vi "P-733 XY Stage Engine.vi"(0 "Notifier Name":string, 11 "Axis Names":string[](array[string])) -> ()   [LabVIEW 2016]
uses:
  Microscope-Control-master/Microscope-Control-master/Device Library/Stages/Stages Controls/Stage Notifier Element.ctl
  Microscope-Control-master/Microscope-Control-master/Device Library/Stages/Stages Controls/Stage Actions.ctl
  Microscope-Control-master/Microscope-Control-master/Device Library/Stages/Stages Controls/Stage Status.ctl
  PI GCS2 DLL/PI_GCS2_DLL_x64.dll
panel:
  out "Success":u32
  in  "Right":bool
  in  "Left":bool
  in  "Y Position (µm)":dbl format="%#.3g"
  in  "Down":bool
  in  "Up":bool
  in  "X Position (µm)":dbl format="%#.3g"
  in  "Step Size (µm)":dbl=0.1
  in  "QUIT":bool
  in  "Abort":bool
  out "P-733 Found":bool
  out "Number Connected":i32
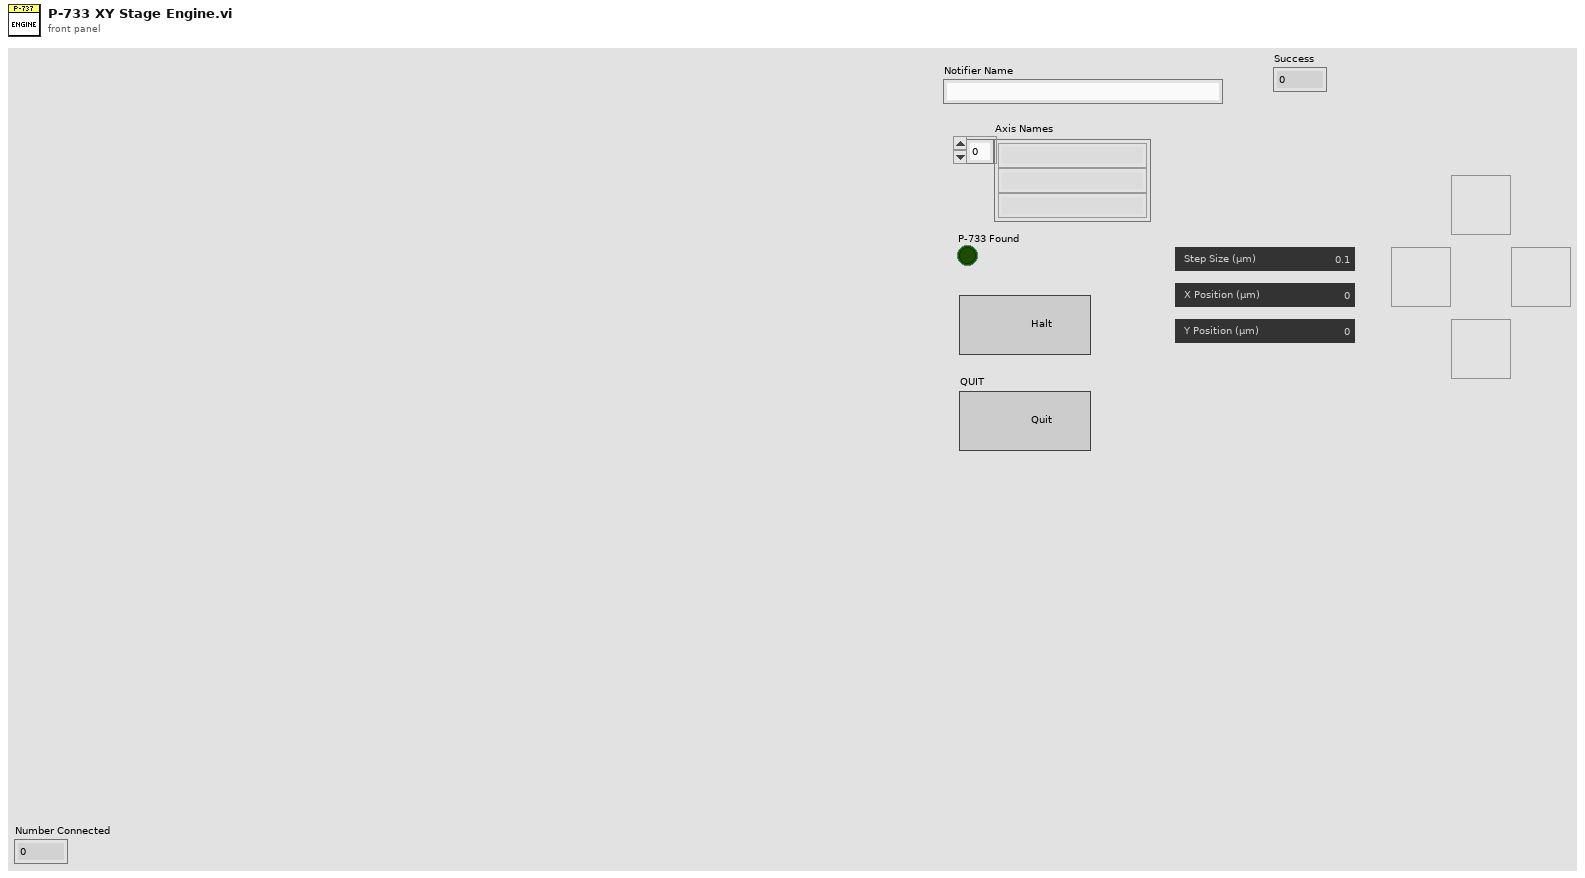
[diagram p1: front panel]
types:
  T1 = typedef "Stage Notifier Element.ctl" = cluster{"Action":T2, "Axis":bool[], "Setpoint":dbl[], "Velocity":dbl, "Cmd Recvd?":bool, "Position":dbl[], "Status":T3, "Misc":variant}
  T2 = typedef "Stage Actions.ctl" = enum16{"Get Position", "MVR", "MOVE", "HALT", "ONTARGET", "ERROR", "REFERENCE", "INIT", "VELOCITY", "STATUS", "EXIT", "HOME", "ZEROPOS", "NANOPOS", "ANALOG", "QUIT"}
  T3 = typedef "Stage Status.ctl" = enum16{"Error", "Abort", "Busy", "On Target"}
  T4 = enum32{"Invalid", "Standard", "Closed", "Hidden", "Minimized", "Maximized"}
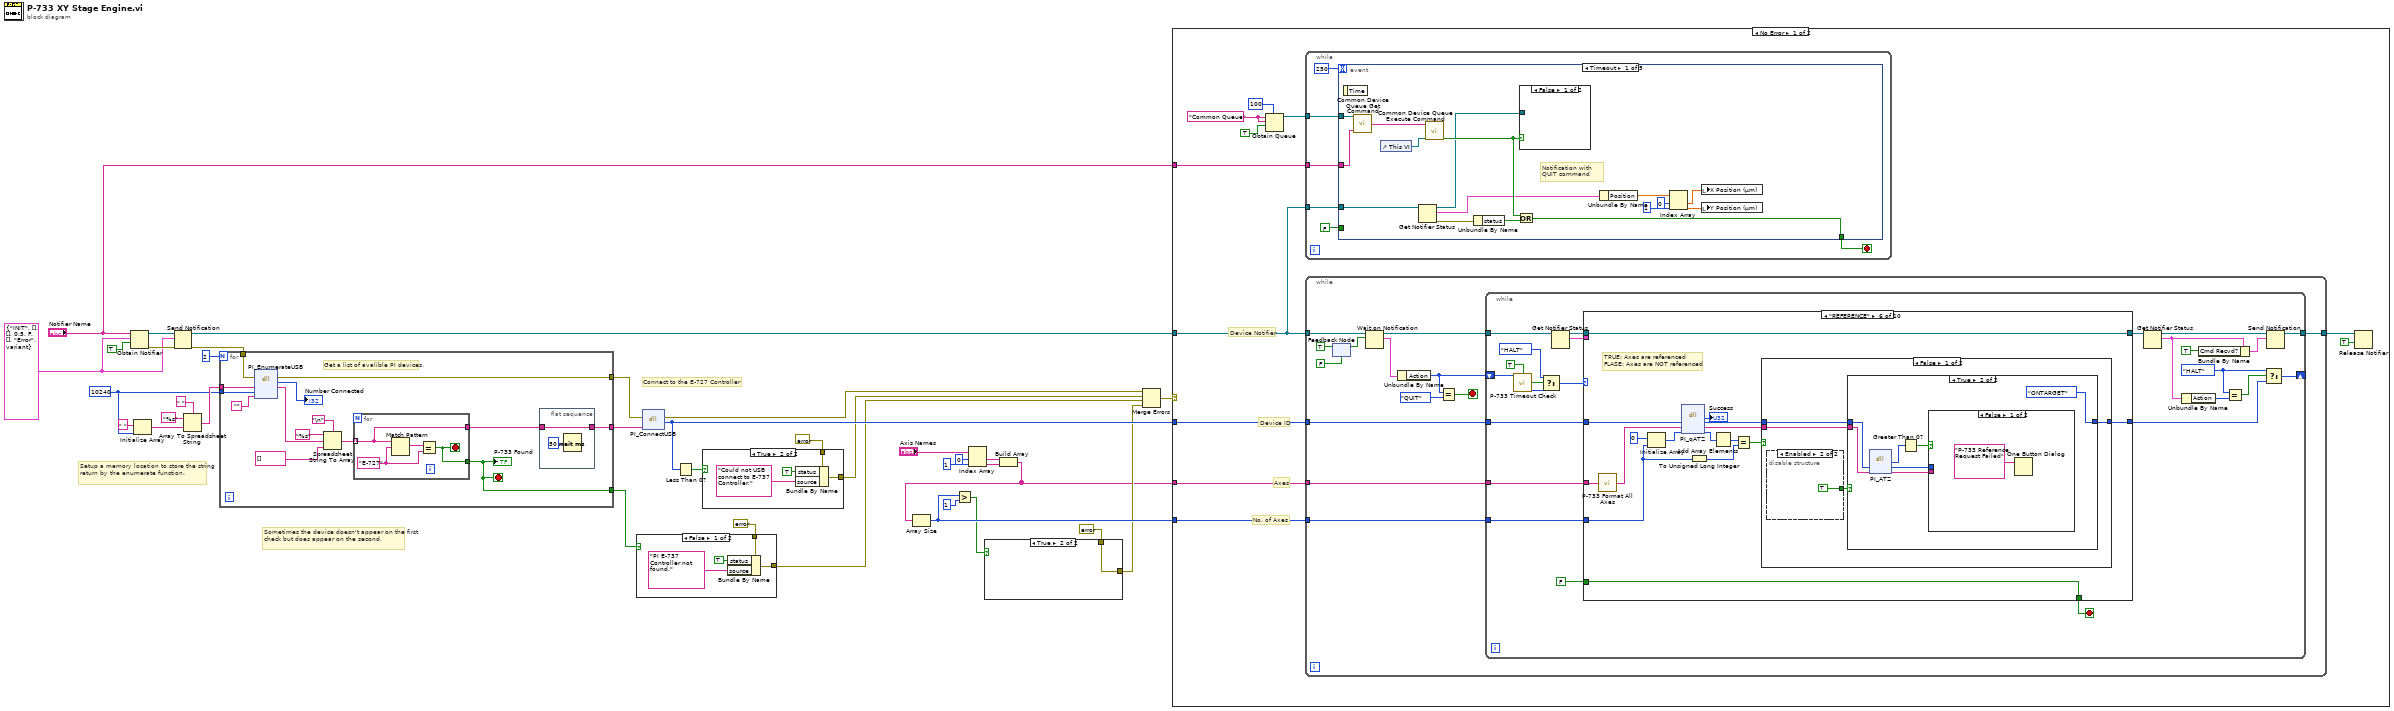
[diagram p0: block diagram]
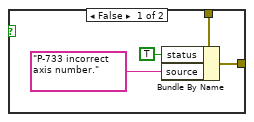
[diagram p2: hidden frame]
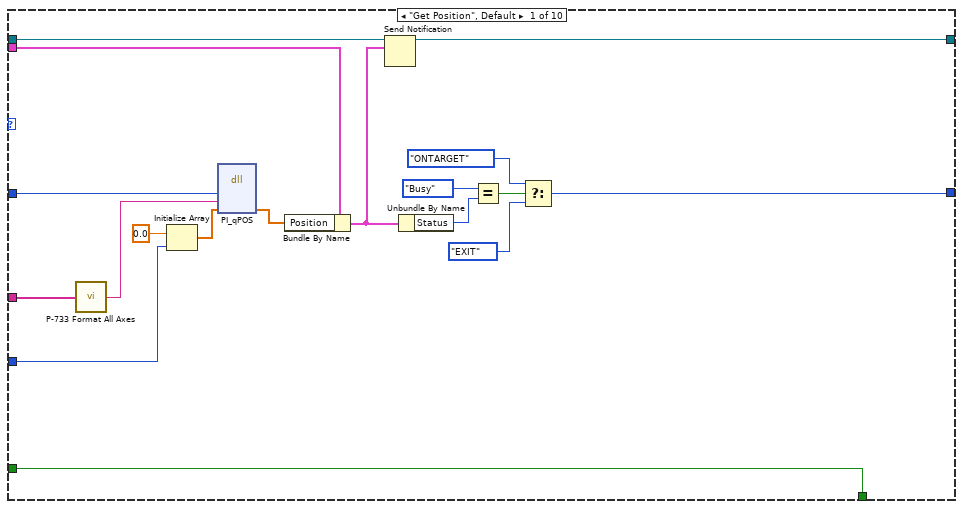
[diagram p5: hidden frame]
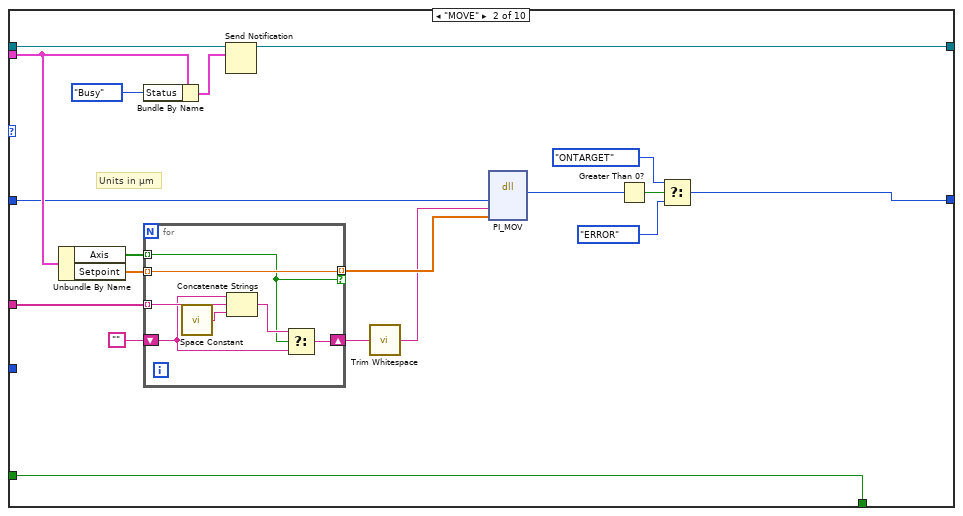
[diagram p6: hidden frame]
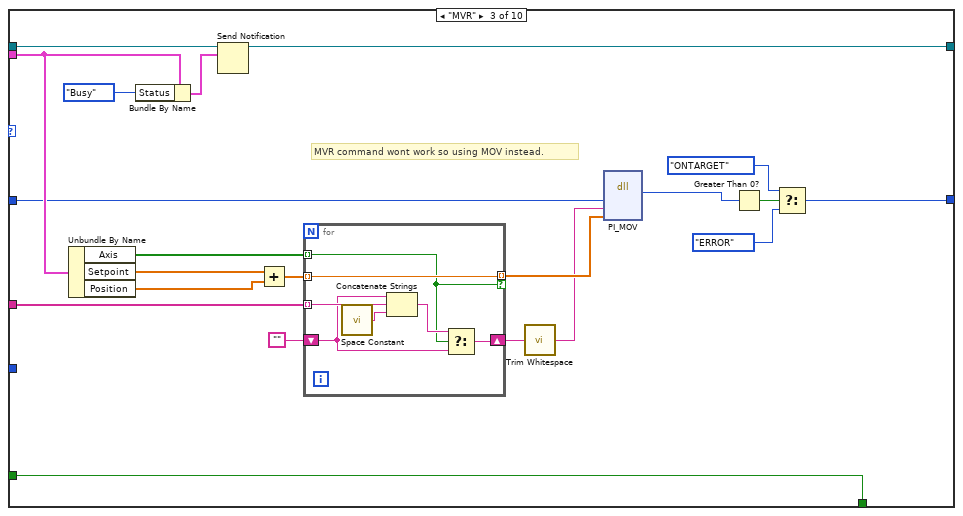
[diagram p7: hidden frame]
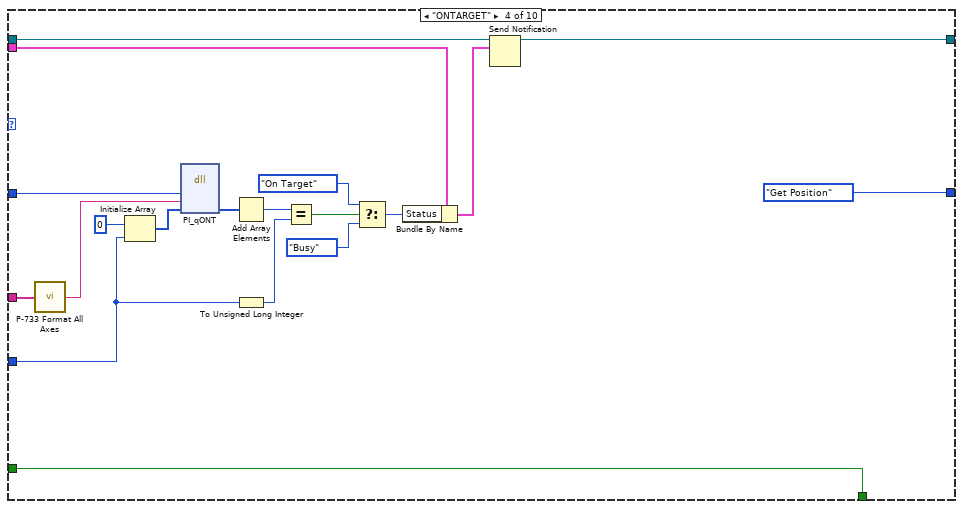
[diagram p8: hidden frame]
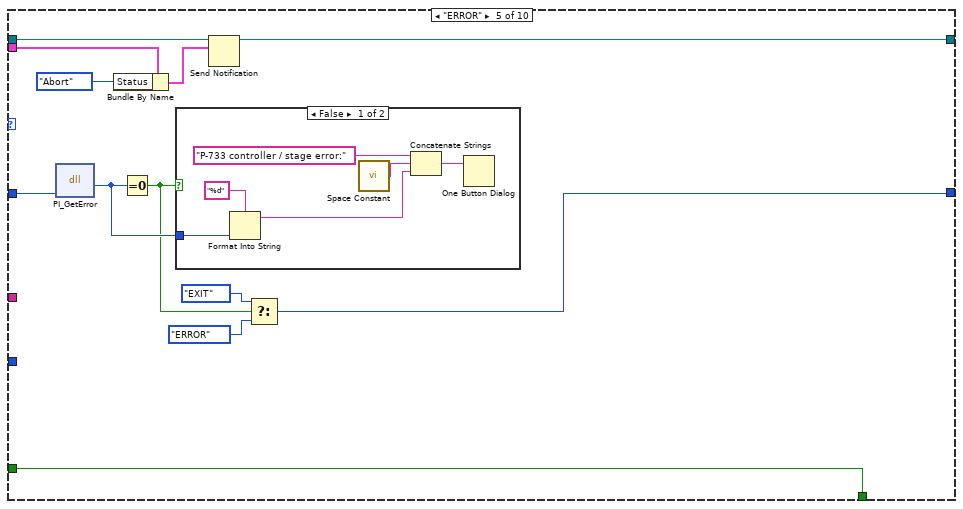
[diagram p9: hidden frame]
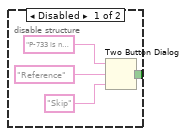
[diagram p11: hidden frame]
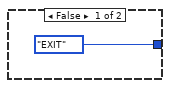
[diagram p12: hidden frame]
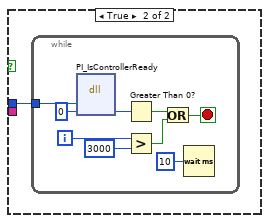
[diagram p13: hidden frame]
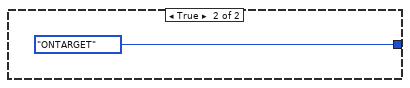
[diagram p14: hidden frame]
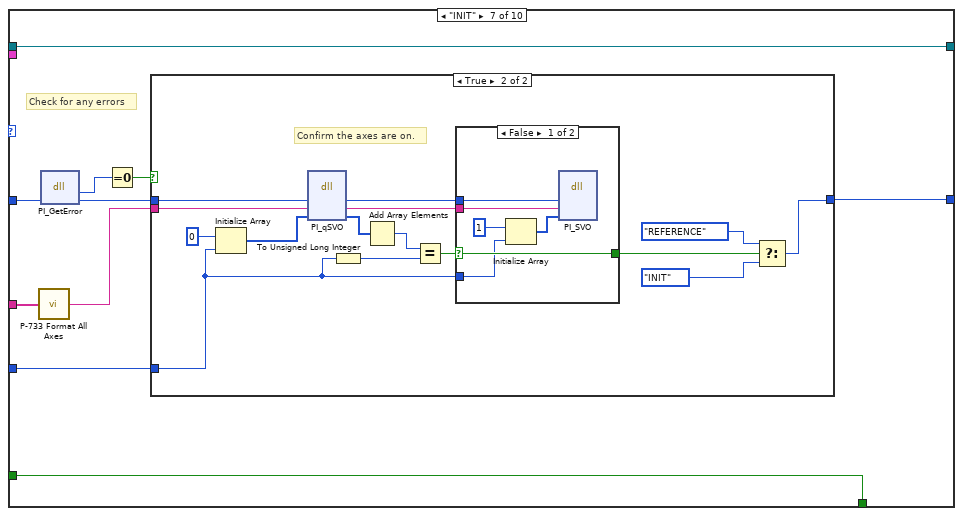
[diagram p15: hidden frame]
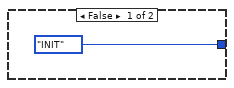
[diagram p16: hidden frame]
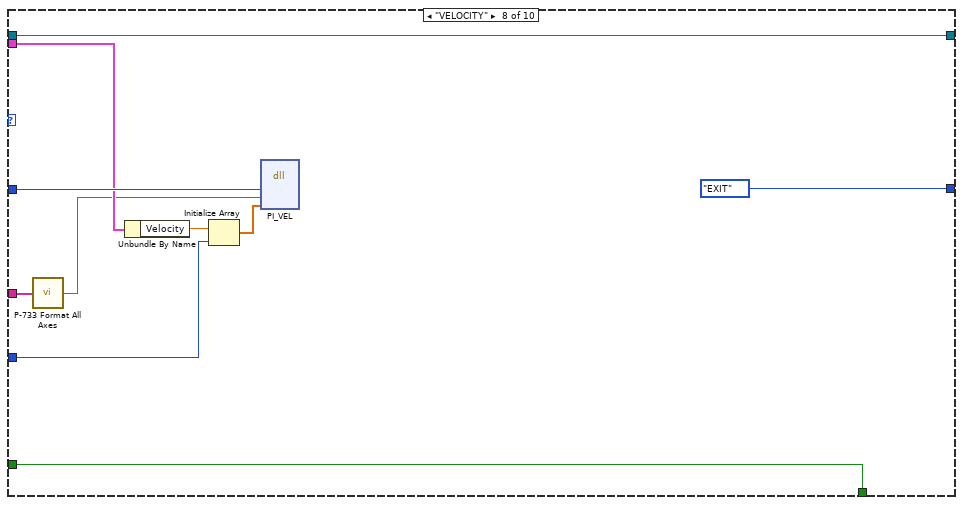
[diagram p18: hidden frame]
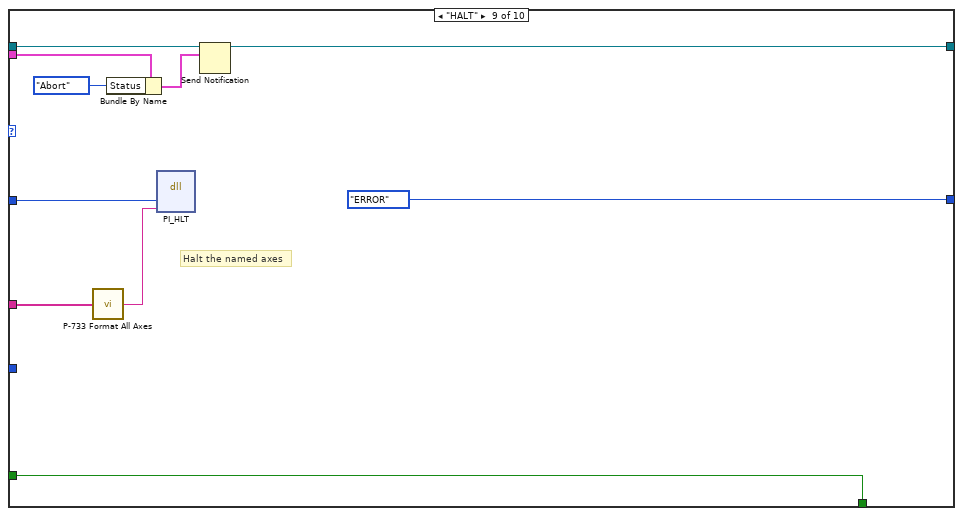
[diagram p19: hidden frame]
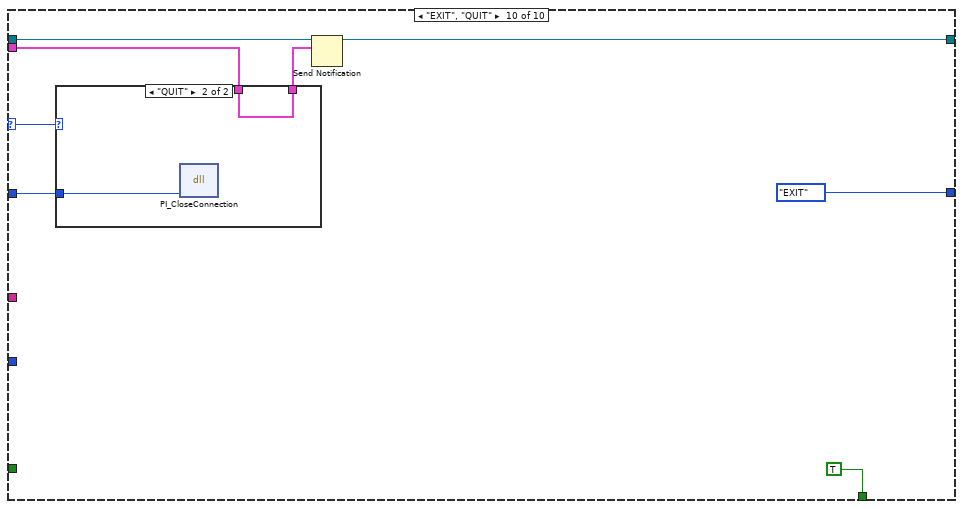
[diagram p20: hidden frame]
diagram:
  w14 = T1 {"Action"=enum."INIT", "Axis"=[], "Setpoint"=[], "Velocity"=0.5, "Cmd Recvd?"=FALSE, "Position"=[], "Status"=enum."Error", "Misc"=variant} ("Stage Status")
  w31 = 10240 ("dimension size")
  # "Setup a memory location to store the string return by the enumerate function."
  # "Connect to the E-727 Controller"
  # "Sometimes the device doesn't appear on the first check but does appear on the second."
  n1 = Obtain Notifier(name (unnamed)="Notifier Name", notification data type=w14, create if not found? (T)=TRUE) -> (notifier out=w17:refnum<notifier>, error out=w16:errorcluster)  [unwired: 1 in, 1 out]
  n2 = Initialize Array(" ", w31) -> (w35:string[])
  n3 = Send Notification(notification=w14, notifier=w17, error in (no error)=w16) -> (notifier out=w13:refnum<notifier>, error out=w15:errorcluster)
  n4 = Array To Spreadsheet String(delimiter (Tab)=" ", array=w35, 3:"%s" ("format string")) -> (spreadsheet string=w32:string)
  n5 = for {
    N: 2 -> [_]
    tunnel: w32 -> [w45]
    tunnel: w31 -> [w44]
    tunnel: [w40] -> w29
    tunnel: [w39] -> w23
    tunnel: [w38] -> w28
    tunnel: w15 -> [w37]
    stop <- w39 stop-if-true
    # "Get a list of avalible PI devices."
    n6 = dll-call lib="C:/Users/Ries Lab/Desktop/4Pi Labview/Microscope-Control/Device Library/Stages/PI/PI GCS2 DLL/PI_GCS2_DLL_x64.dll" fn="PI_EnumerateUSB"(error in=w37, "szBuffer"=w45, "iBufferSize"=w44, "szFilter"="") -> (error out=w38:errorcluster, "return type"=→"Number Connected":i32, "szBuffer"=w42:string)  [unwired: 4 in, 1 out]
    n7 = Spreadsheet String To Array(delimiter (Tab)="\n", format string="%s", spreadsheet string=w42, array type (2D Dbl)=string[] []) -> (array=w47:string[])
    n8 = for {
      tunnel: w47 -> [w54] mode=indexing
      tunnel: [w54] -> w41
      tunnel: [w53] -> w39
      stop <- w53 stop-if-true
      w55 = "E-727"
      n9 = Match Pattern(string=w54, regular expression=w55) -> (match substring=w56:string)  [unwired: 1 in, 3 out]
      n10 = Equal?(x=w56, y=w55) -> (x = y?=w53:bool)
    }
    "P-733 Found" <- w39
    n11 = flat-sequence {
      tunnel: w41 -> [w52]
      tunnel: [w52] -> w40
      frame #0 {
        n12 = Wait (ms)(milliseconds to wait=u32 50) -> ()  [unwired: 1 out]
      }
    }
  }
  n13 = case shown="False" w23 {
    tunnel: errorcluster {"status"=FALSE, "code"=0, "source"=""} ("error in (no error)") -> [w58 w61]
    tunnel: [w57 w61] -> w19
    frame False {
      n14 = Bundle By Name(cluster=w58, "status"=TRUE, "source"="PI E-737 Controller not found.") -> (w57:errorcluster)
    }
    frame True {
    }
  }
  n15 = dll-call lib="C:/Users/Ries Lab/Desktop/4Pi Labview/Microscope-Control/Device Library/Stages/PI/PI GCS2 DLL/PI_GCS2_DLL_x64.dll" fn="PI_ConnectUSB"(error in=w28, "szDescription"=w29) -> (error out=w21:errorcluster, "Device ID"=w26:i32)  [unwired: 3 in, 1 out]
  n16 = Less Than 0?(x=w26) -> (x < 0?=w25:bool)
  n17 = case shown="True" w25 {
    tunnel: errorcluster {"status"=FALSE, "code"=0, "source"=""} ("error in (no error)") -> [w62 w66]
    tunnel: [w62 w63] -> w20
    frame False {
    }
    frame True {
      n18 = Bundle By Name(cluster=w66, "status"=TRUE, "source"="Could not USB connect to E-737 Controller.") -> (w63:errorcluster)
    }
  }
  n19 = Index Array(array="Axis Names", index #1=0 ("index"), index #2=1 ("index")) -> (element #1=w3:string, element #2=w2:string)
  n20 = Build Array(w3, w2) -> (w1:string[])
  n21 = Array Size(array=w1) -> (size(s)=w10:i32)
  n22 = Greater?(x=w10, y=1) -> (0:w8:bool)
  n23 = case shown="True" w8 {
    tunnel: errorcluster {"status"=FALSE, "code"=0, "source"=""} ("error in (no error)") -> [w68 w71]
    tunnel: [w67 w71] -> w7
    frame False {
      n24 = Bundle By Name(cluster=w68, "status"=TRUE, "source"="P-733 incorrect axis number.") -> (w67:errorcluster)
    }
    frame True {
    }
  }
  n25 = Merge Errors(w21, w20, w19, w7) -> (w18:errorcluster)
  n26 = case shown="No Error" w18 {
    selector: w18 -> [_ w434]
    tunnel: w13 -> [w76 w436]
    tunnel: "Notifier Name" -> [w77 _]
    tunnel: w26 -> [w75 w435]
    tunnel: w1 -> [w73 _]
    tunnel: w10 -> [w72 _]
    frame No Error {
      w81 = "Common Queue" ("Unique Notifier Name")
      # "Device Notifier"
      # "No. of Axes"
      # "Axes"
      # "Device ID"
      n27 = Obtain Queue(max queue size (-1, unlimited)=100, name (unnamed)=w81, element data type=w81, create if not found? (T)=TRUE) -> (queue out=w78:refnum<queue>)  [unwired: 1 in, 2 out]
      n28 = while {
        tunnel: w76 -> [w342]
        tunnel: w78 -> [w341]
        tunnel: w77 -> [w340]
        stop <- w343 stop-if-true
        n29 = event shown="[0] Timeout" {
          selector: _ -> [_ _ _ _ _]
          dyn-events: _ -> [_ _ _ _ _]
          timeout: 250 -> [_ _ _ _ _]
          tunnel: [w354 w363 w381 w403 w426] -> w343
          tunnel: w342 -> [w360 _ w374 w395 w429]
          tunnel: w341 -> [w356 _ _ _ _]
          tunnel: w340 -> [w351 _ _ _ _]
          tunnel: FALSE -> [_ w363 w381 w403 w426]
          event Timeout {
            # "Notification with QUIT command"
            n30 = event-data() -> ()  [unwired: 1 in, 1 out]
            n31 = call "Common Device Queue Get Command.vi"("Common Queue"=w356, "Notifier Name"=w351) -> ("Command"=w357:string)  [unwired: 12 in, 1 out]
            n32 = control-ref of="This VI"() -> (w358:refnum<vi>)
            n33 = Get Notifier Status(notifier=w360) -> (notifier out=w352:refnum<notifier>, current notification=w350:T1, error out=w359:errorcluster)  [unwired: 1 in, 2 out]
            n34 = call "Common Device Queue Execute Command.vi"("Common Command"=w357, "VI Refnum"=w358) -> ("Quit?"=w353:bool)  [unwired: 12 in, 1 out]
            n35 = Unbundle By Name(w359) -> ("status"=w355:bool)
            n36 = Or(x=w353, y=w355) -> (x .or. y?=w354:bool)
            n37 = case shown="False" w353 {
              tunnel: w352 -> [_ w362]
              frame False {
              }
              frame True {
                n38 = Send Notification(notification=T1 {"Action"=enum."QUIT", "Axis"=[], "Setpoint"=[], "Velocity"=0.5, "Cmd Recvd?"=FALSE, "Position"=[], "Status"=enum."Error", "Misc"=variant} ("Stage Status"), notifier=w362) -> ()  [unwired: 1 in, 2 out]
              }
            }
            n39 = Unbundle By Name(w350) -> ("Position"=w349:dbl[])
            n40 = Index Array(array=w349, index #1=0 ("index"), index #2=1 ("index")) -> (element #1=w345:dbl, element #2=w346:dbl)
            n41 = local write "X Position (µm)"(w345) -> ()
            n42 = local write "Y Position (µm)"(w346) -> ()
          }
          event Application Instance Close? {
            n43 = event-data() -> ()  [unwired: 1 in, 5 out]
            n44 = control-ref of="This VI"() -> (w365:refnum<vi>)
            n45 = invoke class="VI" method="FP.Open"(reference=w365, "Activate"=TRUE ("Activate?"), "State"=T4."Standard") -> ()  [unwired: 2 in, 5 out]
            n46 = event-data("Discard?"=TRUE) -> ()  [unwired: 1 in, 1 out]
          }
          event "X Position (µm)", "Y Position (µm)": Value Change {
            n47 = event-data() -> ("CtlRef"=w380:refnum<vi>, "NewVal"=w378:dbl)  [unwired: 1 in]
            n48 = Build Array(w378, 0.0) -> (w376:dbl[])
            n49 = property class="DigNum (strict)"(reference=w380) -> ("Label.Text"=w379:string)  [unwired: 1 in, 2 out]
            n50 = case shown="\"Y Position (µm)\"" w379 {
              tunnel: w376 -> [_ w385 w389]
              tunnel: bool[] [TRUE, FALSE] -> [_ w384 w387]
              tunnel: [dbl[] [0.0, 0.0] w385 w388] -> w370
              tunnel: [bool[] [FALSE, FALSE] w384 w386] -> w369
              frame Default {
              }
              frame "X Position (µm)" {
              }
              frame "Y Position (µm)" {
                n51 = Reverse 1D Array(array=w389) -> (reversed array=w388:dbl[])
                n52 = Reverse 1D Array(array=w387) -> (reversed array=w386:bool[])
              }
            }
            n53 = Get Notifier Status(notifier=w374) -> (notifier out=w373:refnum<notifier>, current notification=w372:T1)  [unwired: 1 in, 3 out]
            n54 = Bundle By Name(cluster=w372, "Action"=Stage_Actions."MOVE", "Setpoint"=w370, "Axis"=w369) -> (w368:T1)
            n55 = Send Notification(notification=w368, notifier=w373) -> ()  [unwired: 1 in, 2 out]
          }
          event "Up", "Down", "Left", "Right": Value Change {
            n56 = event-data() -> ("CtlRef"=w398:refnum<vi>)  [unwired: 1 in]
            n57 = property class="Bool"(reference=w398) -> ("Label.Text"=w397:string)  [unwired: 1 in, 2 out]
            n58 = Build Array("Step Size (µm)", 0.0 ("element")) -> (w400:dbl[])
            n59 = case shown="\"Left\", \"Right\"" w397 {
              selector: w397 -> [_ w412 w418]
              tunnel: w400 -> [_ w409 w417]
              tunnel: bool[] [TRUE, FALSE] -> [_ w406 w415]
              tunnel: [dbl[] [0.0, 0.0] w408 w414] -> w392
              tunnel: [bool[] [FALSE, FALSE] w406 w413] -> w391
              frame Default {
              }
              frame "Down", "Up" {
                n60 = Negate(x=w409) -> (-x=w410:dbl[])
                n61 = Equal?(x=w412, y="Down") -> (x = y?=w407:bool)
                n62 = Select(t=w410, s=w407, f=w409) -> (s? t:f=w408:dbl[])
              }
              frame "Left", "Right" {
                n63 = Reverse 1D Array(array=w415) -> (reversed array=w413:bool[])
                n64 = Negate(x=w417) -> (-x=w420:dbl[])
                n65 = Equal?(x=w418, y="Left") -> (x = y?=w419:bool)
                n66 = Select(t=w420, s=w419, f=w417) -> (s? t:f=w416:dbl[])
                n67 = Reverse 1D Array(array=w416) -> (reversed array=w414:dbl[])
              }
            }
            n68 = Get Notifier Status(notifier=w395) -> (notifier out=w396:refnum<notifier>, current notification=w394:T1)  [unwired: 1 in, 3 out]
            n69 = Bundle By Name(cluster=w394, "Action"=Stage_Actions."MVR" ("Actions"), "Setpoint"=w392, "Axis"=w391) -> (w390:T1)
            n70 = Send Notification(notification=w390, notifier=w396) -> ()  [unwired: 1 in, 2 out]
          }
          event "QUIT", "Abort": Value Change {
            n71 = event-data() -> ("CtlRef"=w428:refnum<vi>)  [unwired: 1 in]
            n72 = property class="Bool"(reference=w428) -> ("Label.Text"=w427:string)  [unwired: 1 in, 2 out]
            n73 = case shown="\"Abort\"" w427 {
              tunnel: [Stage_Actions."EXIT" ("Action") Stage_Actions."QUIT" ("Action") Stage_Actions."HALT" ("Action")] -> w425
              frame "Default", Default {
              }
              frame "QUIT" {
              }
              frame "Abort" {
              }
            }
            n74 = Get Notifier Status(notifier=w429) -> (notifier out=w423:refnum<notifier>, current notification=w422:T1)  [unwired: 1 in, 3 out]
            n75 = Bundle By Name(cluster=w422, "Action"=w425) -> (w424:T1)
            n76 = Send Notification(notification=w424, notifier=w423) -> ()  [unwired: 1 in, 2 out]
          }
        }
      }
      n77 = while {
        tunnel: w76 -> [w94]
        tunnel: w75 -> [w93]
        tunnel: [w91] -> w74
        tunnel: w73 -> [w89]
        tunnel: w72 -> [w88]
        stop <- w90 stop-if-true
        n78 = feedback #1(FALSE) -> (w84:bool)
        n79 = feedback-in #1(TRUE ("ignore previous (F)")) -> ()
        n80 = Wait on Notification(notifier=w94, ignore previous (F)=w84) -> (notifier out=w83:refnum<notifier>, notification=w92:T1)  [unwired: 2 in, 2 out]
        n81 = Unbundle By Name(w92) -> ("Action"=w87:T2)
        n82 = Equal?(x=w87, y=Stage_Actions."QUIT") -> (x = y?=w90:bool)
        n83 = while {
          tunnel: w93 -> [w118]
          tunnel: w83 -> [w115]
          shift-right: [w117] -> _
          shift-left: w87 -> [w111]
          tunnel: [w97] -> w91
          tunnel: w89 -> [w105]
          tunnel: w88 -> [w106]
          stop <- w119 stop-if-true
          w102 = Stage_Actions."HALT" ("t")
          n84 = call "P-733 Timeout Check.vi"("Action"=w111, "User Input?"=TRUE) -> ("Timeout?"=w110:bool, "Action (Dup)"=w109:T2)  [unwired: 12 in]
          n85 = Select(t=Stage_Actions."HALT" ("y"), s=w110, f=w109) -> (s? t:f=w108:T2)
          n86 = Get Notifier Status(notifier=w115) -> (notifier out=w114:refnum<notifier>, current notification=w113:T1)  [unwired: 1 in, 3 out]
          n87 = case shown="\"REFERENCE\"" w108 {
            selector: w108 -> [_ _ _ _ _ _ _ _ _ w333]
            tunnel: w114 -> [w123 w141 w170 w195 w216 w245 w278 w317 w325 w331]
            tunnel: FALSE -> [w135 w157 w185 w211 w223 w244 w282 w316 w318 _]
            tunnel: [w135 w157 w185 w211 w223 w244 w282 w316 w318 TRUE] -> w119
            tunnel: [w129 w153 w181 Stage_Actions."Get Position" ("y") w217 w240 w279 Stage_Actions."EXIT" ("y") Stage_Actions."ERROR" ("y") Stage_Actions."EXIT" ("y")] -> w116
            tunnel: w118 -> [w136 w150 w178 w210 w222 w243 w284 w315 w327 w334]
            tunnel: [w121 w139 w168 w193 w215 w245 w278 w317 w323 w329] -> w104
            tunnel: w113 -> [w128 w151 w179 w201 w214 _ _ w314 w326 w332]
            tunnel: w106 -> [w127 _ _ w205 _ w236 w275 w310 _ _]
            tunnel: w105 -> [w125 w146 w175 w197 _ w232 w277 w312 w321 _]
            frame "Get Position", Default {
              n88 = call "P-733 Format All Axes.vi"("All Axis Array"=w125) -> ("All Axes String"=w124:string)  [unwired: 14 in]
              n89 = Initialize Array(0.0 ("element"), w127) -> (w138:dbl[])
              n90 = dll-call lib="C:/Users/Ries Lab/Desktop/4Pi Labview/Microscope-Control/Device Library/Stages/PI/PI GCS2 DLL/PI_GCS2_DLL_x64.dll" fn="PI_qPOS"("Device ID"=w136, "szAxes"=w124, "pdValueArray"=w138) -> ("pdValueArray"=w126:dbl[])  [unwired: 6 in, 2 out]
              n91 = Bundle By Name(cluster=w128, "Position"=w126) -> (w122:T1)
              n92 = Send Notification(notification=w122, notifier=w123) -> (notifier out=w121:refnum<notifier>)  [unwired: 1 in, 1 out]
              n93 = Unbundle By Name(w122) -> ("Status"=w134:T3)
              n94 = Equal?(x=Stage_Status."Busy", y=w134) -> (x = y?=w132:bool)
              n95 = Select(t=Stage_Actions."ONTARGET" ("y"), s=w132, f=Stage_Actions."EXIT" ("y")) -> (s? t:f=w129:T2)
            }
            frame "MOVE" {
              # "Units in µm"
              n96 = Unbundle By Name(w151) -> ("Axis"=w148:bool[], "Setpoint"=w147:dbl[])
              n97 = Bundle By Name(cluster=w151, "Status"=Stage_Status."Busy") -> (w140:T1)
              n98 = for {
                tunnel: w148 -> [w160] mode=indexing
                tunnel: w147 -> [w161] mode=indexing
                tunnel: w146 -> [w164] mode=indexing
                shift-right: [w159] -> w143
                shift-left: "" -> [w158]
                tunnel: [w161] -> w144 mode=indexing if=w160
                n99 = call <vilib>:"Space Constant.vi"() -> ("String"=w163:string)
                n100 = Concatenate Strings(w158, w164, w163) -> (w162:string)
                n101 = Select(t=w162, s=w160, f=w158) -> (s? t:f=w159:string)
              }
              n102 = Send Notification(notification=w140, notifier=w141) -> (notifier out=w139:refnum<notifier>)  [unwired: 1 in, 1 out]
              n103 = call <vilib>:"Trim Whitespace.vi"("string"=w143) -> ("trimmed string"=w142:string)  [unwired: 1 in]
              n104 = dll-call lib="C:/Users/Ries Lab/Desktop/4Pi Labview/Microscope-Control/Device Library/Stages/PI/PI GCS2 DLL/PI_GCS2_DLL_x64.dll" fn="PI_MOV"("Device ID"=w150, "szAxes"=w142, "pdValueArray"=w144) -> ("Success"=w149:u32)  [unwired: 6 in, 2 out]
              n105 = Greater Than 0?(x=w149) -> (x > 0?=w156:bool)
              n106 = Select(t=Stage_Actions."ONTARGET" ("Action"), s=w156, f=Stage_Actions."ERROR" ("Action")) -> (s? t:f=w153:T2)
            }
            frame "MVR" {
              # "MVR command wont work so using MOV instead."
              n107 = Unbundle By Name(w179) -> ("Axis"=w176:bool[], "Setpoint"=w165:dbl[], "Position"=w167:dbl[])
              n108 = Bundle By Name(cluster=w179, "Status"=Stage_Status."Busy") -> (w169:T1)
              n109 = Send Notification(notification=w169, notifier=w170) -> (notifier out=w168:refnum<notifier>)  [unwired: 1 in, 1 out]
              n110 = Add(x=w165, y=w167) -> (x+y=w166:dbl[])
              n111 = for {
                tunnel: w176 -> [w188] mode=indexing
                tunnel: w166 -> [w189] mode=indexing
                tunnel: w175 -> [w192] mode=indexing
                shift-right: [w187] -> w172
                shift-left: "" -> [w186]
                tunnel: [w189] -> w173 mode=indexing if=w188
                n112 = call <vilib>:"Space Constant.vi"() -> ("String"=w191:string)
                n113 = Concatenate Strings(w186, w192, w191) -> (w190:string)
                n114 = Select(t=w190, s=w188, f=w186) -> (s? t:f=w187:string)
              }
              n115 = call <vilib>:"Trim Whitespace.vi"("string"=w172) -> ("trimmed string"=w171:string)  [unwired: 1 in]
              n116 = dll-call lib="C:/Users/Ries Lab/Desktop/4Pi Labview/Microscope-Control/Device Library/Stages/PI/PI GCS2 DLL/PI_GCS2_DLL_x64.dll" fn="PI_MOV"("Device ID"=w178, "szAxes"=w171, "pdValueArray"=w173) -> ("Success"=w177:u32)  [unwired: 6 in, 2 out]
              n117 = Greater Than 0?(x=w177) -> (x > 0?=w184:bool)
              n118 = Select(t=Stage_Actions."ONTARGET" ("Action"), s=w184, f=Stage_Actions."ERROR" ("Action")) -> (s? t:f=w181:T2)
            }
            frame "ONTARGET" {
              n119 = call "P-733 Format All Axes.vi"("All Axis Array"=w197) -> ("All Axes String"=w196:string)  [unwired: 14 in]
              n120 = Initialize Array(u32 0 ("element"), w205) -> (w208:u32[])
              n121 = dll-call lib="C:/Users/Ries Lab/Desktop/4Pi Labview/Microscope-Control/Device Library/Stages/PI/PI GCS2 DLL/PI_GCS2_DLL_x64.dll" fn="PI_qONT"("Device ID"=w210, "szAxes"=w196, "pdValueArray"=w208) -> ("pdValueArray"=w207:u32[])  [unwired: 6 in, 2 out]
              n122 = Add Array Elements(numeric array=w207) -> (sum=w206:u32)
              n123 = To Unsigned Long Integer(number=w205) -> (unsigned 32bit integer=w204:u32)
              n124 = Equal?(x=w206, y=w204) -> (x = y?=w203:bool)
              n125 = Select(t=Stage_Status."On Target" ("Status"), s=w203, f=Stage_Status."Busy" ("Status")) -> (s? t:f=w198:T3)
              n126 = Bundle By Name(cluster=w201, "Status"=w198) -> (w194:T1)
              n127 = Send Notification(notification=w194, notifier=w195) -> (notifier out=w193:refnum<notifier>)  [unwired: 1 in, 1 out]
            }
            frame "ERROR" {
              n128 = dll-call lib="C:/Users/Ries Lab/Desktop/4Pi Labview/Microscope-Control/Device Library/Stages/PI/PI GCS2 DLL/PI_GCS2_DLL_x64.dll" fn="PI_GetError"("Device ID"=w222) -> ("Error Code"=w221:i32)  [unwired: 4 in, 2 out]
              n129 = Bundle By Name(cluster=w214, "Status"=Stage_Status."Abort") -> (w213:T1)
              n130 = Equal To 0?(x=w221) -> (x = 0?=w220:bool)
              n131 = case shown="False" w220 {
                tunnel: w221 -> [w227 _]
                frame False {
                  n132 = Format Into String(format string="%d", w227) -> (resulting string=w225:string)  [unwired: 2 in, 1 out]
                  n133 = call <vilib>:"Space Constant.vi"() -> ("String"=w228:string)
                  n134 = Concatenate Strings("P-733 controller / stage error:", w228, w225) -> (w224:string)
                  n135 = One Button Dialog(message=w224) -> ()  [unwired: 1 in, 1 out]
                }
                frame True {
                }
              }
              n136 = Send Notification(notification=w213, notifier=w216) -> (notifier out=w215:refnum<notifier>)  [unwired: 1 in, 1 out]
              n137 = Select(t=Stage_Actions."EXIT", s=w220, f=Stage_Actions."ERROR" ("Action")) -> (s? t:f=w217:T2)
            }
            frame "REFERENCE" {
              # "TRUE: Axes are referenced\nFLASE: Axes are NOT referenced"
              n138 = call "P-733 Format All Axes.vi"("All Axis Array"=w232) -> ("All Axes String"=w231:string)  [unwired: 14 in]
              n139 = Initialize Array(u32 0 ("element"), w236) -> (w241:u32[])
              n140 = dll-call lib="C:/Users/Ries Lab/Desktop/4Pi Labview/Microscope-Control/Device Library/Stages/PI/PI GCS2 DLL/PI_GCS2_DLL_x64.dll" fn="PI_qATZ"("Device ID"=w243, "szAxes"=w231, "pdValueArray"=w241) -> ("Success"=→"Success":u32, "Device ID"=w238:i32, "szAxes"=w239:string, "pdValueArray"=w237:u32[])  [unwired: 3 in, 2 out]
              n141 = To Unsigned Long Integer(number=w236) -> (unsigned 32bit integer=w234:u32)
              n142 = Add Array Elements(numeric array=w237) -> (sum=w235:u32)
              n143 = Equal?(x=w235, y=w234) -> (x = y?=w233:bool)
              n144 = case shown="False" w233 {
                tunnel: [w246 Stage_Actions."ONTARGET" ("Action")] -> w240
                tunnel: w239 -> [w247 _]
                tunnel: w238 -> [w248 _]
                frame False {
                  n145 = disable-structure shown="Enabled" {
                    disable-tunnel: [w251 TRUE ("T button?")] -> w249
                    frame Disabled {
                      n146 = Two Button Dialog(message="P-733 is not referenced.", 1:"Skip" ("F button name (\"Cancel\")"), 2:"Reference" ("T button name (\"OK\")")) -> (T button?=w251:bool)
                    }
                    frame Enabled {
                    }
                  }
                  n147 = case shown="True" w249 {
                    tunnel: w248 -> [_ w256]
                    tunnel: w247 -> [_ w257]
                    tunnel: [Stage_Actions."EXIT" ("Action") Stage_Actions."ONTARGET" ("Action")] -> w246
                    frame False {
                    }
                    frame True {
                      n148 = dll-call lib="C:/Users/Ries Lab/Desktop/4Pi Labview/Microscope-Control/Device Library/Stages/PI/PI GCS2 DLL/PI_GCS2_DLL_x64.dll" fn="PI_ATZ"("Device ID"=w256, "szAxes"=w257) -> ("Success"=w258:u32, "Device ID"=w260:i32, "szAxes"=w261:string)  [unwired: 3 in, 2 out]
                      n149 = Greater Than 0?(x=w258) -> (x > 0?=w259:bool)
                      n150 = case shown="False" w259 {
                        tunnel: w260 -> [_ w264]
                        tunnel: w261 -> [_ _]
                        frame False {
                          n151 = One Button Dialog(message="P-733 Reference Request Failed") -> ()  [unwired: 1 in, 1 out]
                        }
                        frame True {
                          n152 = while {
                            tunnel: w264 -> [w273]
                            i -> [w271]
                            stop <- w266 stop-if-true
                            n153 = dll-call lib="C:/Users/Ries Lab/Desktop/4Pi Labview/Microscope-Control/Device Library/Stages/PI/PI GCS2 DLL/PI_GCS2_DLL_x64.dll" fn="PI_IsControllerReady"("Device ID"=w273, "piControllerReady"=0) -> ("piControllerReady"=w269:i32)  [unwired: 5 in, 2 out]
                            n154 = Greater Than 0?(x=w269) -> (x > 0?=w268:bool)
                            n155 = Greater?(x=w271, y=3000) -> (0:w267:bool)
                            n156 = Or(x=w268, y=w267) -> (x .or. y?=w266:bool)
                            n157 = Wait (ms)(milliseconds to wait=u32 10) -> ()  [unwired: 1 out]
                          }
                        }
                      }
                    }
                  }
                }
                frame True {
                }
              }
            }
            frame "INIT" {
              # "Check for any errors"
              n158 = call "P-733 Format All Axes.vi"("All Axis Array"=w277) -> ("All Axes String"=w276:string)  [unwired: 14 in]
              n159 = dll-call lib="C:/Users/Ries Lab/Desktop/4Pi Labview/Microscope-Control/Device Library/Stages/PI/PI GCS2 DLL/PI_GCS2_DLL_x64.dll" fn="PI_GetError"("Device ID"=w284) -> ("Error Code"=w283:i32, "Device ID"=w280:i32)  [unwired: 3 in, 2 out]
              n160 = Equal To 0?(x=w283) -> (x = 0?=w281:bool)
              n161 = case shown="True" w281 {
                tunnel: w280 -> [_ w300]
                tunnel: w276 -> [_ w299]
                tunnel: [Stage_Actions."INIT" ("Action") w297] -> w279
                tunnel: w275 -> [_ w292]
                frame False {
                }
                frame True {
                  # "Confirm the axes are on."
                  n162 = Initialize Array(u32 0 ("element"), w292) -> (w294:u32[])
                  n163 = dll-call lib="C:/Users/Ries Lab/Desktop/4Pi Labview/Microscope-Control/Device Library/Stages/PI/PI GCS2 DLL/PI_GCS2_DLL_x64.dll" fn="PI_qSVO"("Device ID"=w300, "szAxes"=w299, "pdValueArray"=w294) -> ("Device ID"=w290:i32, "szAxes"=w291:string, "pdValueArray"=w289:u32[])  [unwired: 4 in, 2 out]
                  n164 = To Unsigned Long Integer(number=w292) -> (unsigned 32bit integer=w286:u32)
                  n165 = Add Array Elements(numeric array=w289) -> (sum=w288:u32)
                  n166 = Equal?(x=w288, y=w286) -> (x = y?=w287:bool)
                  n167 = case shown="False" w287 {
                    selector: w287 -> [w304 w307]
                    tunnel: w291 -> [w305 _]
                    tunnel: w290 -> [w306 _]
                    tunnel: [w304 w307] -> w298
                    tunnel: w292 -> [w302 _]
                    frame False {
                      n168 = Initialize Array(u32 1 ("element"), w302) -> (w301:u32[])
                      n169 = dll-call lib="C:/Users/Ries Lab/Desktop/4Pi Labview/Microscope-Control/Device Library/Stages/PI/PI GCS2 DLL/PI_GCS2_DLL_x64.dll" fn="PI_SVO"("Device ID"=w306, "szAxes"=w305, "pdValueArray"=w301) -> ()  [unwired: 7 in, 2 out]
                    }
                    frame True {
                    }
                  }
                  n170 = Select(t=Stage_Actions."REFERENCE" ("Action"), s=w298, f=Stage_Actions."INIT" ("Action")) -> (s? t:f=w297:T2)
                }
              }
            }
            frame "VELOCITY" {
              n171 = call "P-733 Format All Axes.vi"("All Axis Array"=w312) -> ("All Axes String"=w308:string)  [unwired: 14 in]
              n172 = Unbundle By Name(w314) -> ("Velocity"=w311:dbl)
              n173 = Initialize Array(w311, w310) -> (w309:dbl[])
              n174 = dll-call lib="C:/Users/Ries Lab/Desktop/4Pi Labview/Microscope-Control/Device Library/Stages/PI/PI GCS2 DLL/PI_GCS2_DLL_x64.dll" fn="PI_VEL"("Device ID"=w315, "szAxes"=w308, "pdValueArray"=w309) -> ()  [unwired: 7 in, 2 out]
            }
            frame "HALT" {
              # "Halt the named axes"
              n175 = call "P-733 Format All Axes.vi"("All Axis Array"=w321) -> ("All Axes String"=w319:string)  [unwired: 14 in]
              n176 = Bundle By Name(cluster=w326, "Status"=Stage_Status."Abort") -> (w324:T1)
              n177 = dll-call lib="C:/Users/Ries Lab/Desktop/4Pi Labview/Microscope-Control/Device Library/Stages/PI/PI GCS2 DLL/PI_GCS2_DLL_x64.dll" fn="PI_HLT"("Device ID"=w327, "szAxes"=w319) -> ()  [unwired: 6 in, 2 out]
              n178 = Send Notification(notification=w324, notifier=w325) -> (notifier out=w323:refnum<notifier>)  [unwired: 1 in, 1 out]
            }
            frame "EXIT", "QUIT" {
              n179 = case shown="\"QUIT\"" w333 {
                tunnel: w334 -> [_ w337]
                tunnel: w332 -> [w336 w338]
                tunnel: [w336 w338] -> w330
                frame Default {
                }
                frame "QUIT" {
                  n180 = dll-call lib="C:/Users/Ries Lab/Desktop/4Pi Labview/Microscope-Control/Device Library/Stages/PI/PI GCS2 DLL/PI_GCS2_DLL_x64.dll" fn="PI_CloseConnection"("Device ID"=w337) -> ()  [unwired: 5 in, 2 out]
                }
              }
              n181 = Send Notification(notification=w330, notifier=w331) -> (notifier out=w329:refnum<notifier>)  [unwired: 1 in, 1 out]
            }
          }
          n182 = Get Notifier Status(notifier=w104) -> (notifier out=w98:refnum<notifier>, current notification=w96:T1)  [unwired: 1 in, 3 out]
          n183 = Unbundle By Name(w96) -> ("Action"=w103:T2)
          n184 = Bundle By Name(cluster=w96, "Cmd Recvd?"=TRUE) -> (w99:T1)
          n185 = Equal?(x=w102, y=w103) -> (x = y?=w101:bool)
          n186 = Select(t=w102, s=w101, f=w116) -> (s? t:f=w117:T2)
          n187 = Send Notification(notification=w99, notifier=w98) -> (notifier out=w97:refnum<notifier>)  [unwired: 1 in, 1 out]
        }
      }
      n188 = Release Notifier(notifier=w74, force destroy? (F)=TRUE) -> ()  [unwired: 1 in, 3 out]
    }
    frame Error {
      n189 = dll-call lib="C:/Users/Ries Lab/Desktop/4Pi Labview/Microscope-Control/Device Library/Stages/PI/PI GCS2 DLL/PI_GCS2_DLL_x64.dll" fn="PI_CloseConnection"(error in=w434, "Device ID"=w435) -> (error out=w433:errorcluster)  [unwired: 4 in, 1 out]
      n190 = Release Notifier(notifier=w436, force destroy? (F)=TRUE, error in (no error)=w433) -> (error out=w441:errorcluster)  [unwired: 2 out]
      n191 = Unbundle By Name(w441) -> ("source"=w438:string)
      n192 = Concatenate Strings("P-733 Initialization Error", "\r", w438) -> (w437:string)
      n193 = One Button Dialog(message=w437) -> ()  [unwired: 1 in, 1 out]
    }
  }
